vi "Shutdown.vi"(8 "error in":errorcluster, 11 "Oven in":refnum<class "Oven.lvclass">) -> (0 "error out":errorcluster, 3 "Oven out":refnum<class "Oven.lvclass">)   [LabVIEW 2018, in "Oven.lvlib" / "Oven.lvclass"]
uses:
  Oven.lvclass
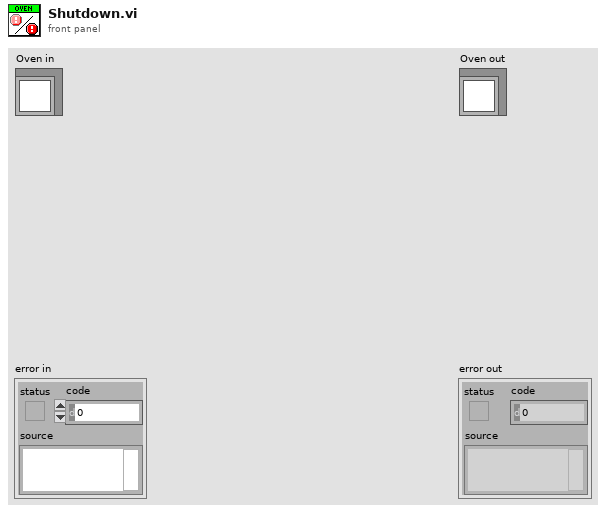
[diagram p1: front panel]
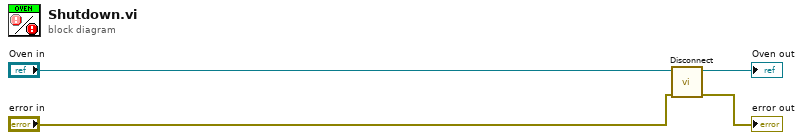
[diagram p0: block diagram]
diagram:
  n1 = call-dynamic "Disconnect.vi"("error in (no error)"="error in", "Oven in"="Oven in") -> ("error out"=→"error out":errorcluster, "Oven out"=→"Oven out":refnum<class "Oven.lvclass">)  [unwired: 8 in]
